vi "Remove.vi"(8 "error in (no error)":errorcluster, 10 "Key":string, 11 "Array In":refnum<class "Array.lvclass">) -> (0 "error out":errorcluster, 1 "Value":refnum<class>, 3 "Array Out":refnum<class "Array.lvclass">)   [LabVIEW 2013, in "LapDog.Collections.v_.Maps.Implementations.lvlib" / "Array.lvclass"]
doc: "Removes the key-value pair from the collection.\n\nIf the key does not exist, error 510203 is returned."
uses:
  Array.lvclass
  Array.lvclass/Array.ctl
  LapDog.Collections.Common/LapDog.Collections.v_.Common.lvlib
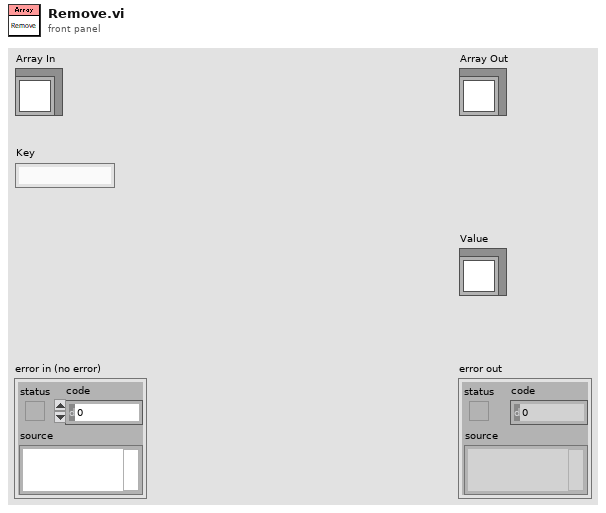
[diagram p1: front panel]
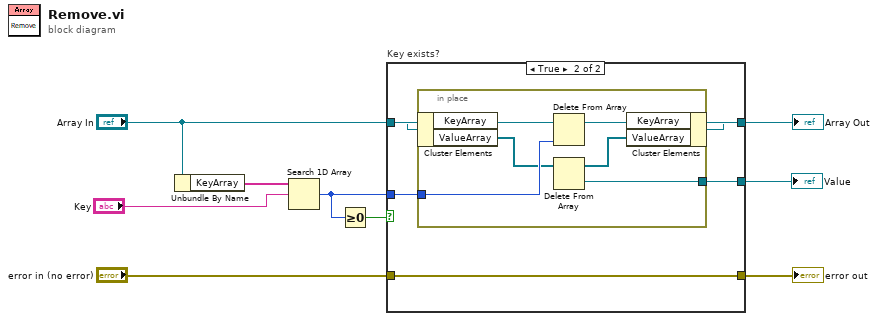
[diagram p0: block diagram]
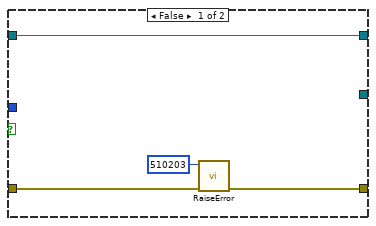
[diagram p2: hidden frame]
diagram:
  n1 = Unbundle By Name("Array In") -> ("KeyArray"=w8:string[])
  n2 = Search 1D Array(1D array=w8, element="Key") -> (index of element=w6:i32)  [unwired: 1 in]
  n3 = Greater Or Equal To 0?(x=w6) -> (x >= 0?=w7:bool)
  n4 = case "Key exists?" shown="True" w7 {
    tunnel: [w12 w15] -> _
    tunnel: "Array In" -> [w12 w16]
    tunnel: "error in (no error)" -> [w11 w17]
    tunnel: [w10 w17] -> w2
    tunnel: w6 -> [_ w14]
    tunnel: [_ w13] -> w1
    frame False {
      n5 = call "RaiseError.vi"("error in (no error)"=w11, "Error Code"=510203) -> ("error out"=w10:errorcluster)  [unwired: 9 in]
    }
    frame True {
      n6 = in-place {
        in-place-border: w14 -> [w21]
        in-place-border: [w18] -> w13
        n7 = in-place-cluster #1(w16) -> ("KeyArray"=w23:string[], "ValueArray"=w20:refnum<class>[])
        n8 = Delete From Array(array=w23, index=w21) -> (array with subset deleted=w22:string[])  [unwired: 1 in, 1 out]
        n9 = Delete From Array(array=w20) -> (deleted portion=w18:refnum<class>, array with subset deleted=w19:refnum<class>[])  [unwired: 2 in]
        n10 = in-place-cluster #1("KeyArray"=w22, "ValueArray"=w19) -> (w15:refnum<class "Array.lvclass">)
      }
    }
  }
  "error out" <- w2
  "Value" <- w1
  "Array Out" <- "Array In"
